vi "LIA_FPGA-host.vi"(0 "dec1":i16=1, 1 "dec2":i16=1, 3 "Ref Signal":fxp<+/-,16,16>, 4 "stages":i8=1, 5 "decimation":i16=1024, 7 "nominal freq  (LIA)":fxp<+,16,0>=0.010009765625, 8 "Filter Constant":i64, 9 "While Loop Counter":i16, 10 "K":fxp<+,16,0>=0.001007080078125, 11 "Sampling Frequency":i32) -> (2 "f":fxp<+/-,32,0> format="%.32g", 6 "F graph":fxp<+,64,64>, 12 "Degree":fxp<+,1,1>, 13 "sig":i16 format="%.0x", 14 "phase (pi)":fxp<+/-,16,2>, 15 "K Constant":fxp<+/-,32,16>, 17 "f PLL Output":i64, 18 "Nominal Freq":fxp<+/-,64,32>, 19 "R":fxp<+,1,1>)   [LabVIEW 2012]
uses:
  <vilib>/rvi/DataTransferAndStorage/Container/Common/niFpgaContainerMetaDataKey.ctl
  <vilib>/rvi/DataTransferAndStorage/Container/Common/niFpgaContainerState.ctl
  <vilib>/rvi/DataTransferAndStorage/Container/Common/niFpgaDataTypeControl.ctl
  <vilib>/rvi/DataTransferAndStorage/Container/Common/niFpgaContainerImplementationControl.ctl
  <vilib>/rvi/DataTransferAndStorage/Container/Common/niFpgaContainerArbitrationOptionsControl.ctl
  <vilib>/rvi/DataTransferAndStorage/Container/Common/niFpgaTransferTypeControl.ctl
  <vilib>/rvi/DataTransferAndStorage/Container/Common/niFpgaContainerInitializationParameters.ctl
  <vilib>/rvi/Memory/Memory_Types/niFpgaMemoryInterfaceConfiguration.ctl
  <vilib>/rvi/FIFO/Fifo_Types/niFpgaFifoControlLogicControl.ctl
  <vilib>/rvi/FXPMathLib/FxpDiv/subVIs/nifxpmath_Div_SimConfig.ctl
  <vilib>/rvi/FXPMathLib/FxpRectToPolar/subVIs/nifxpmath_RectToPolar_SimConfig.ctl
  <vilib>/rvi/DataTransferAndStorage/Container/Common/niFpgaContainerGetUniqueNameForEmu.vi
  <vilib>/rvi/DataTransferAndStorage/Container/Common/niFpgaContainerSetEmuInfo.vi
  <vilib>/rvi/eio/common/nirviEmuReportErrorAndStop.vi
  <vilib>/rvi/eio/common/nirviEmuTemplateMethod_errors.vi
  <vilib>/rvi/Emulation/niFpgaSctlEmulationGetInTimedLoop.vi
  <vilib>/rvi/FIFO/Fifo_Resource/nirvififoEmulationSetSize.vi
  <vilib>/rvi/Emulation/niFpgaSctlEmulationFifoFullMgr.vi
  <vilib>/rvi/errors/niFpgaSetErrorForExecOnDevCompSimple.vi
  <vilib>/rvi/FXPMathLib/FxpDiv/simVIs/DllFxpDivTemp_sub.vi
  <vilib>/rvi/FXPMathLib/FxpRectToPolar/simVIs/DllFxpRectToPolarTemp_sub.vi
  <vilib>/rvi/Emulation/niFpgaSctlEmulationResourceMgr.vi
  <vilib>/rvi/LocalResourceManager/LocalResourceManager.xnode
  <vilib>/rvi/FXPMathLib/FxpInterpret/XNode/nifxpmath_Interpret.xnode
  <vilib>/eio/EIONode/EIONode.xnode
  <vilib>/rvi/FXPMathLib/FxpMul/XNode/nifxpmath_Multiplier.xnode
  <vilib>/rvi/DataTransferAndStorage/Container/XNode/niFpgaContainer.xnode
  <vilib>/rvi/FIFO/Fifo_Resource/nirvififoEmulationRead.vi
  <vilib>/rvi/FXPMathLib/FxpDiv/XNode/nifxpmath_Div.xnode
  <vilib>/rvi/FXPMathLib/FxpRectToPolar/XNode/nifxpmath_RectToPolar.xnode
  <vilib>/rvi/FIFO/Fifo_Resource/nirvififoEmulationWrite.vi
  <vilib>/rvi/FXPMathLib/sim/FxpSim.dll
panel:
  out "Period1":fxp<+/-,16,16>
  out "ref":i16 format="%.0x"
  out "channelQ":i64
  out "channelI":i64
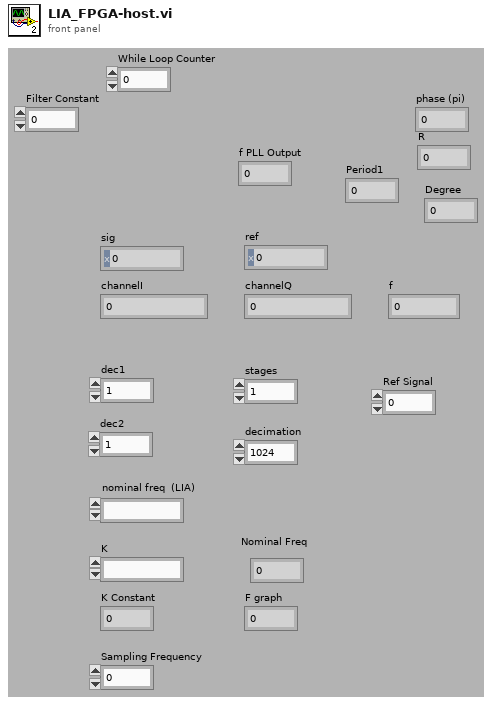
[diagram p1: front panel]
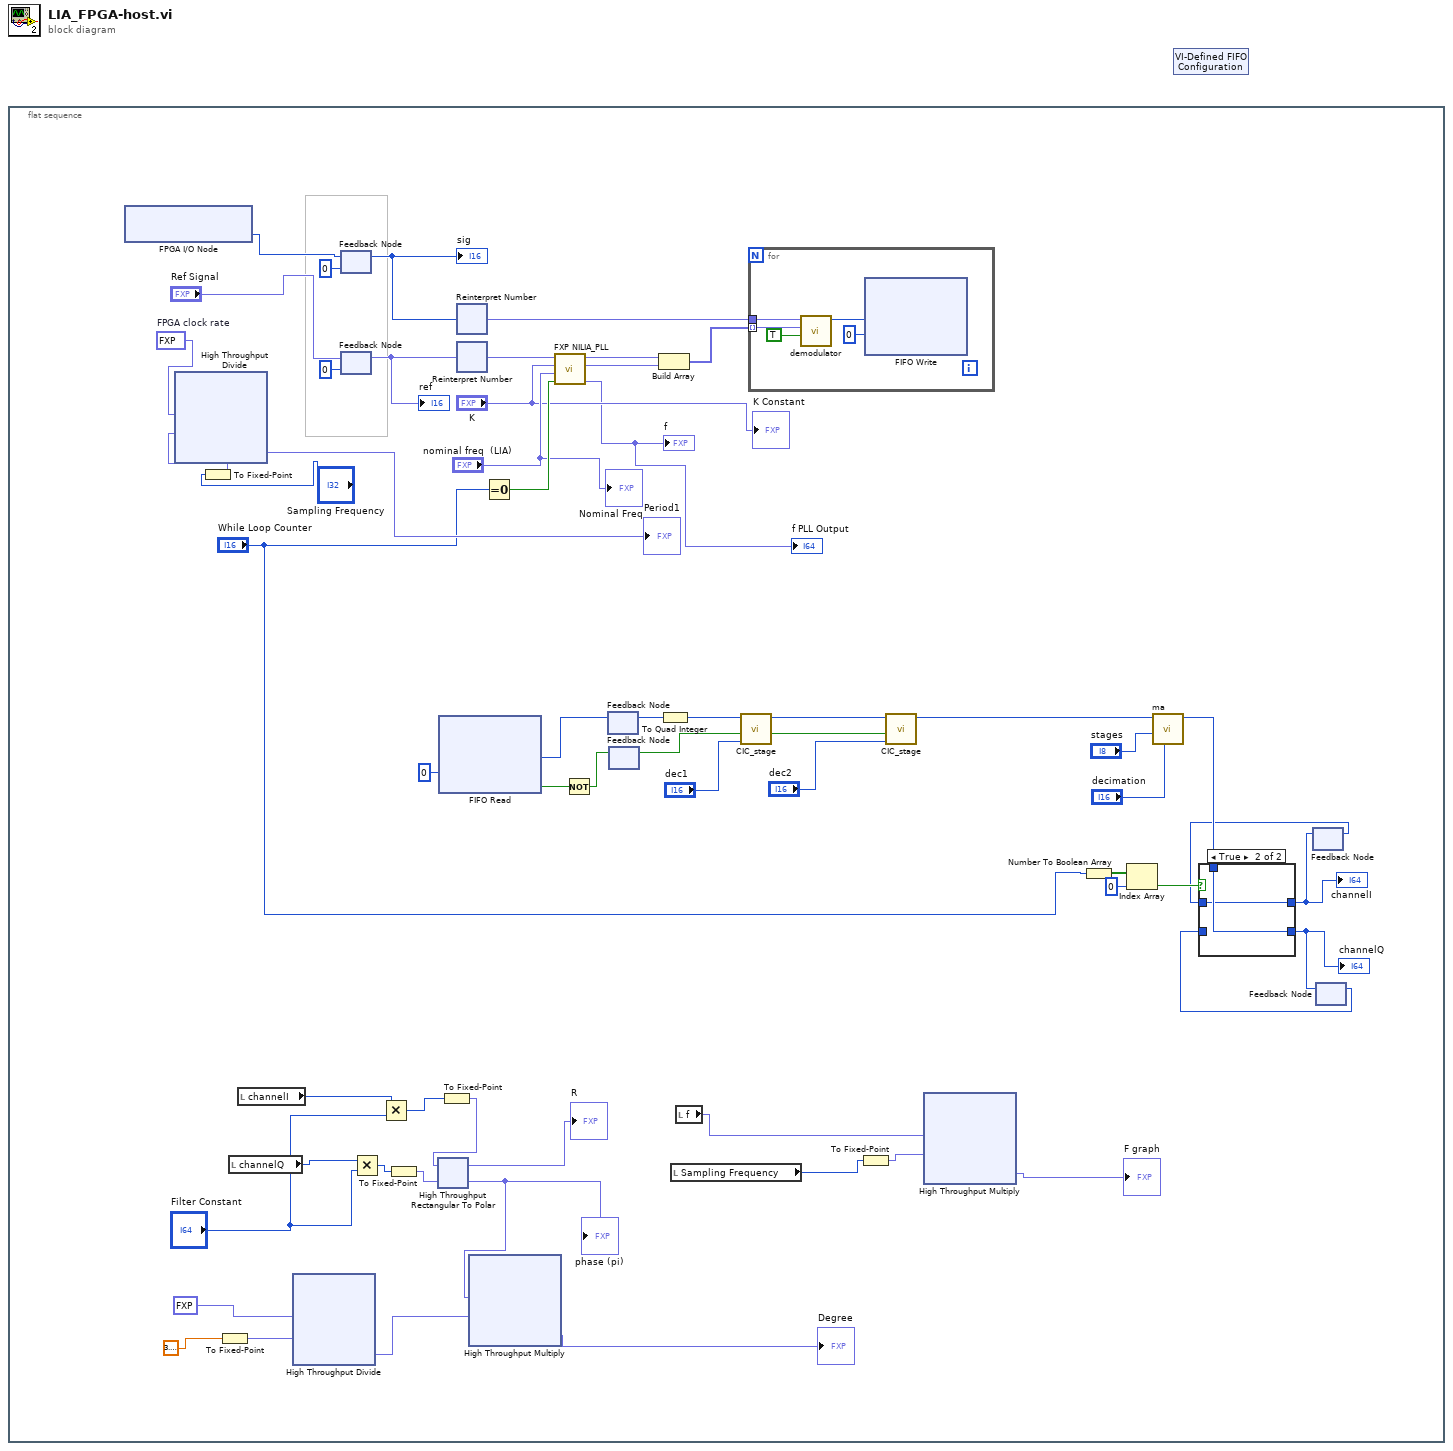
[diagram p0: block diagram]
diagram:
  n1 = flat-sequence {
    frame #0 {
      w48 = fxp<+,17,26> 40000000.0  # FPGA clock rate
      n2 = xnode "FPGA I/O Node"() -> ("Connector0/AI7"=w43:i16)  [unwired: 1 in, 1 out]
      n3 = To Fixed-Point(number="Sampling Frequency") -> (fixed-point=w45:fxp<+/-,32,32>)  [unwired: 1 in]
      n4 = xnode "High Throughput Divide"("x"=w48, "y"=w45) -> ("x/y"=→"Period1":fxp<+/-,27,27>)
      n5 = To Fixed-Point(number=sgl 3.1415927) -> (fixed-point=w18:fxp<+/-,64,64>)  [unwired: 1 in]
      n6 = local read "channelQ"() -> (w29:i64)
      n7 = local read "channelI"() -> (w30:i64)
      n8 = xnode "High Throughput Divide"("x"=fxp<+,6,8> 180.0, "y"=w18) -> ("x/y"=w20:fxp<+/-,9,9>)
      n9 = feedback #1(i16 0 ("y")) -> (w56:i16)
      "sig" <- w56
      n10 = feedback-in #1(w43) -> ()
      n11 = feedback #2(i16 0 ("z [I32.1]")) -> (w55:fxp<+/-,16,16>)
      "ref" <- w55
      n12 = feedback-in #2("Ref Signal") -> ()
      n13 = Multiply(x=w29, y="Filter Constant") -> (x*y=w25:i64)
      n14 = Multiply(x=w30, y="Filter Constant") -> (x*y=w27:i64)
      n15 = To Fixed-Point(number=w25) -> (fixed-point=w24:fxp<+/-,64,64>)  [unwired: 1 in]
      n16 = xnode ("FIFO Read")("Timeout"=0) -> ("Element"=w10:i32, "Timed Out?"=w9:bool)  [unwired: 1 in, 1 out]
      n17 = To Fixed-Point(number=w27) -> (fixed-point=w26:fxp<+/-,64,64>)  [unwired: 1 in]
      n18 = xnode "High Throughput Rectangular To Polar"("x"=w26, "y"=w24) -> ("magnitude"=→"R":fxp<+,64,64>, "phase (pi)"=w21:fxp<+/-,16,2>)
      "phase (pi)" <- w21
      n19 = xnode "Reinterpret Number"("x"=w56) -> ("y"=w59:fxp<+/-,16,1>)
      n20 = xnode "Reinterpret Number"("x"=w55) -> ("y"=w54:fxp<+/-,16,1>)
      n21 = xnode "High Throughput Multiply"("x"=w21, "y"=w20) -> ("x*y"=→"Degree":fxp<+/-,25,11>)
      n22 = Equal To 0?(x="While Loop Counter") -> (x = 0?=w51:bool)
      n23 = call "FXP NILIA_PLL.vi"("reset?"=w51, "norminal freq [U16.0]"="nominal freq  (LIA)", "alpha [U16.0]"="K", "x[I16.1]"=w54) -> ("f"=→"f" →"f PLL Output":fxp<+/-,32,0>, "sin(z)"=w53:fxp<+/-,16,2>, "cos(z)"=w52:fxp<+/-,16,2>)  [unwired: 4 in, 1 out]
      n24 = Not(x=w9) -> (.not. x?=w8:bool)
      n25 = feedback #3() -> (w12:i32)  [unwired: 1 out]
      n26 = feedback-in #3(w10) -> ()
      n27 = feedback #4() -> (w6:bool)  [unwired: 1 out]
      n28 = feedback-in #4(w8) -> ()
      n29 = Build Array(w52, w53) -> (w60:fxp<+/-,16,2>[])
      n30 = To Quad Integer(1:w12) -> (0:w7:i64)
      n31 = local read "Sampling Frequency"() -> (w15:i32)
      n32 = local read "f"() -> (w14:fxp<+/-,32,0>)
      n33 = call "CIC_stage.vi"("decimate factor"="dec1", "New Data"=w6, "input"=w7) -> ("Data Ready"=w4:bool, "output"=w5:i64)  [unwired: 7 out]
      n34 = for {
        tunnel: w59 -> [w158]
        tunnel: w60 -> [w156] mode=indexing
        n35 = call "demodulator.vi"("New Data"=TRUE, "ref"=w156, "signal"=w158) -> ("x*y"=w159:i32)  [unwired: 8 out]
        n36 = xnode ("FIFO Write")("Element"=w159, "Timeout"=0) -> ()  [unwired: 1 in, 2 out]
      }
      n37 = To Fixed-Point(number=w15) -> (fixed-point=w16:fxp<+/-,32,32>)  [unwired: 1 in]
      n38 = call "CIC_stage.vi"("decimate factor"="dec2", "New Data"=w4, "input"=w5) -> ("output"=w40:i64)  [unwired: 8 out]
      n39 = xnode "High Throughput Multiply"("x"=w14, "y"=w16) -> ("x*y"=→"F graph":fxp<+/-,64,32>)
      n40 = Number To Boolean Array(number="While Loop Counter") -> (Boolean array=w39:bool[])
      n41 = Index Array "Index Array"(array=w39, index=0) -> (element=w37:bool)
      n42 = call "ma.vi"("decimate"="decimation", "stages"="stages", "input"=w40) -> ("output"=w36:i64)  [unwired: 8 out]
      n43 = feedback #5() -> (w33:i64)  [unwired: 1 in]
      n44 = feedback #6() -> (w32:i64)  [unwired: 1 in]
      n45 = case shown="True" w37 {
        tunnel: w36 -> [w126 w128]
        tunnel: [w126 w127] -> w34
        tunnel: [w125 w128] -> w35
        tunnel: w33 -> [_ w127]
        tunnel: w32 -> [w125 _]
        frame False {
        }
        frame True {
        }
      }
      "channelI" <- w34
      "channelQ" <- w35
      n46 = feedback-in #5(w34) -> ()
      n47 = feedback-in #6(w35) -> ()
      "Nominal Freq" <- "nominal freq  (LIA)"
      "K Constant" <- "K"
    }
  }
  n48 = xnode "VI-Defined FIFO Configuration"() -> ()  [unwired: 1 out]
